vi "Get Value (Value[]).vi"(8 "error in (no error)":errorcluster, 10 "Keys":string[](array[string]), 11 "JSON Value in":refnum<class "JSON Value.lvclass">) -> (0 "error out":errorcluster, 2 "JSON Value out":refnum<class "JSON Value.lvclass">)   [LabVIEW 2016, in "JSON Value.lvclass"]
uses:
  JSON Value.lvclass
  subVIs/Errors.ctl
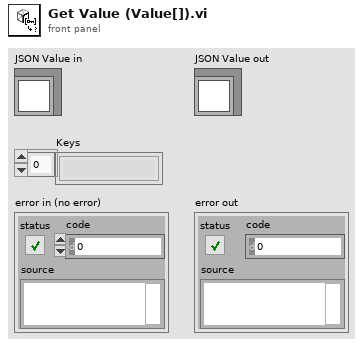
[diagram p1: front panel]
types:
  T1 = typedef "JSON Value.lvclass/Errors.ctl" = enum16{"No key", "Key path type", "Array OOB", "Type Mismatch", "Invalid Token"}
  T2 = typedef "JSON Value.lvclass/JSON Types.ctl" = enum16{"String", "Numeric", "Boolean", "NULL", "Object", "Array"}
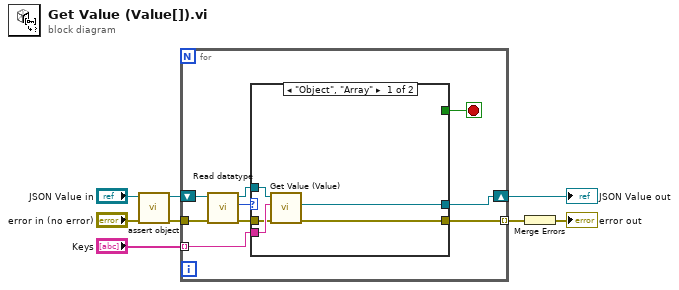
[diagram p0: block diagram]
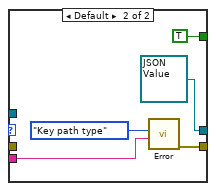
[diagram p2: hidden frame]
diagram:
  n1 = call "assert object.vi"("error in (no error)"="error in (no error)", "JSON Value in"="JSON Value in") -> ("error out"=w3:errorcluster, "JSON Value out"=w1:refnum<class "JSON Value.lvclass">)  [unwired: 8 in]
  n2 = for {
    tunnel: "Keys" -> [w17] mode=indexing
    shift-right: [w16] -> w7
    shift-left: w1 -> [w13]
    tunnel: w3 -> [w10]
    tunnel: [w15] -> w5 mode=indexing
    stop <- w14 stop-if-true
    n3 = call "Read datatype.vi"("error in (no error)"=w10, "JSON Value in"=w13) -> ("error out"=w11:errorcluster, "datatype"=w9:T2, "JSON Value out"=w12:refnum<class "JSON Value.lvclass">)  [unwired: 7 in]
    n4 = case shown="\"Object\", \"Array\"" w9 {
      tunnel: w17 -> [w22 w24]
      tunnel: [w21 refnum<class "JSON Value.lvclass"> refnum ("JSON out")] -> w16
      tunnel: w12 -> [w18 _]
      tunnel: [w19 w26] -> w15
      tunnel: w11 -> [w20 _]
      tunnel: [_ TRUE] -> w14
      frame "Object", "Array" {
        n5 = call "Get Value (Value).vi"("error in (no error)"=w20, "key"=w22, "JSON Value in"=w18) -> ("error out"=w19:errorcluster, "JSON Value out"=w21:refnum<class "JSON Value.lvclass">)  [unwired: 7 in]
      }
      frame Default {
        n6 = call "Error.vi"("Data"=w24, 9:Errors."Key path type") -> ("error out"=w26:errorcluster)  [unwired: 8 in]
      }
    }
  }
  "JSON Value out" <- w7
  n7 = Merge Errors(w5) -> (→"error out":errorcluster)
